vi "DeviceManager.vi"() -> ()   [LabVIEW 2017]
uses:
  D:/upwork/Laser Measurement Tool/Laser/tests/KIM101/Thorlabs.MotionControl.DeviceManagerCLI.dll
  Thorlabs.MotionControl.DeviceManagerCLI.dll
panel:
  out "IsDeviceConnected":bool
  in  "serialNo":string="97000001"
  out "error out":errorcluster
  out "Device List":string[](array[string])
  out "GetDeviceListSize":i16
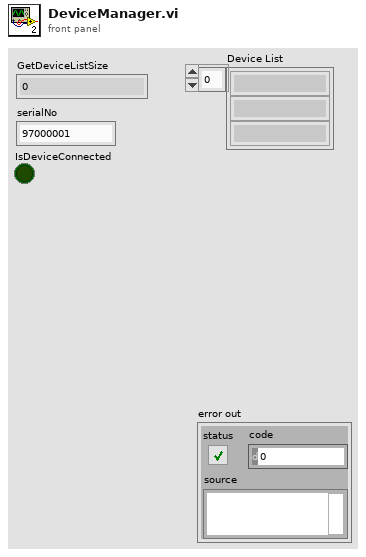
[diagram p1: front panel]
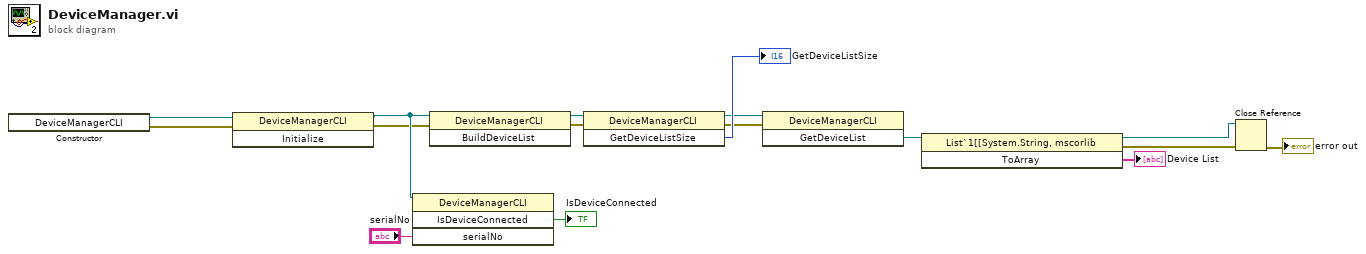
[diagram p0: block diagram]
diagram:
  n1 = constructor class="DeviceManagerCLI"() -> (reference out=w2:refnum<k24>, error out=w1:errorcluster)  [unwired: 3 in, 1 out]
  n2 = invoke class="DeviceManagerCLI" method="Initialize"(reference=w2, error in=w1) -> (reference out=w4:refnum<k24>, error out=w3:errorcluster)  [unwired: 1 in, 1 out]
  n3 = invoke class="DeviceManagerCLI" method="IsDeviceConnected"(reference=w4, "serialNo"="serialNo") -> ("IsDeviceConnected"=→"IsDeviceConnected":bool)  [unwired: 2 in, 3 out]
  n4 = invoke class="DeviceManagerCLI" method="BuildDeviceList"(reference=w4, error in=w3) -> (reference out=w16:refnum<k24>, error out=w14:errorcluster)  [unwired: 1 in, 1 out]
  n5 = invoke class="DeviceManagerCLI" method="GetDeviceListSize"(reference=w16, error in=w14) -> (reference out=w13:refnum<k24>, error out=w12:errorcluster, "GetDeviceListSize"=→"GetDeviceListSize":i16)  [unwired: 1 in]
  n6 = invoke class="DeviceManagerCLI" method="GetDeviceList"(reference=w13, error in=w12) -> ("GetDeviceList"=w11:refnum<k24>)  [unwired: 1 in, 2 out]
  n7 = invoke class="List`1[[System.String, mscorlib" method="ToArray"(reference=w11) -> (reference out=w9:refnum<k24>, error out=w8:errorcluster, "ToArray"=→"Device List":string[])  [unwired: 2 in]
  n8 = Close Reference(reference=w9, error in (no error)=w8) -> (error out=→"error out":errorcluster)
